vi "Get_TTL_pulse_length_at_input_2_and_start.vi"(9 "TTL pulse length to trigger start, ms":dbl=300.0, 10 "ReadStatus in":refnum<notifier>, 11 "VISA resource name":refnum<visa-resource-name>="ASRL3::INSTR") -> (0 "Start acquisition":bool, 1 "Measured TTL pulse length":dbl=0.41002368927001953, 2 "ReadStatus out":refnum<notifier>, 3 "VISA resource name out":refnum<visa-resource-name>="ASRL3::INSTR")   [LabVIEW 2016]
panel:
  out "TTL pulse start time":timestamp=timestamp(3602496054.061625 s since 1904-01-01)
  in  "TTL pulse started":bool
  out "Notifier error out":errorcluster
  out "VISA error out":errorcluster={"status"=FALSE, "code"=1073676294, "source"="VISA Read in Stream_data.vi->Get_TTL_pulse_length_at_input_2.vi"}
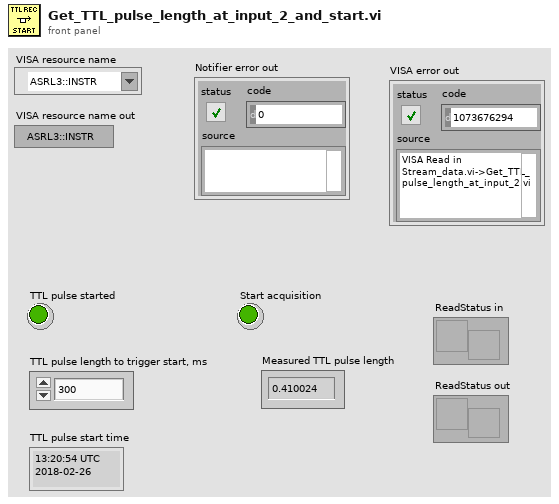
[diagram p1: front panel]
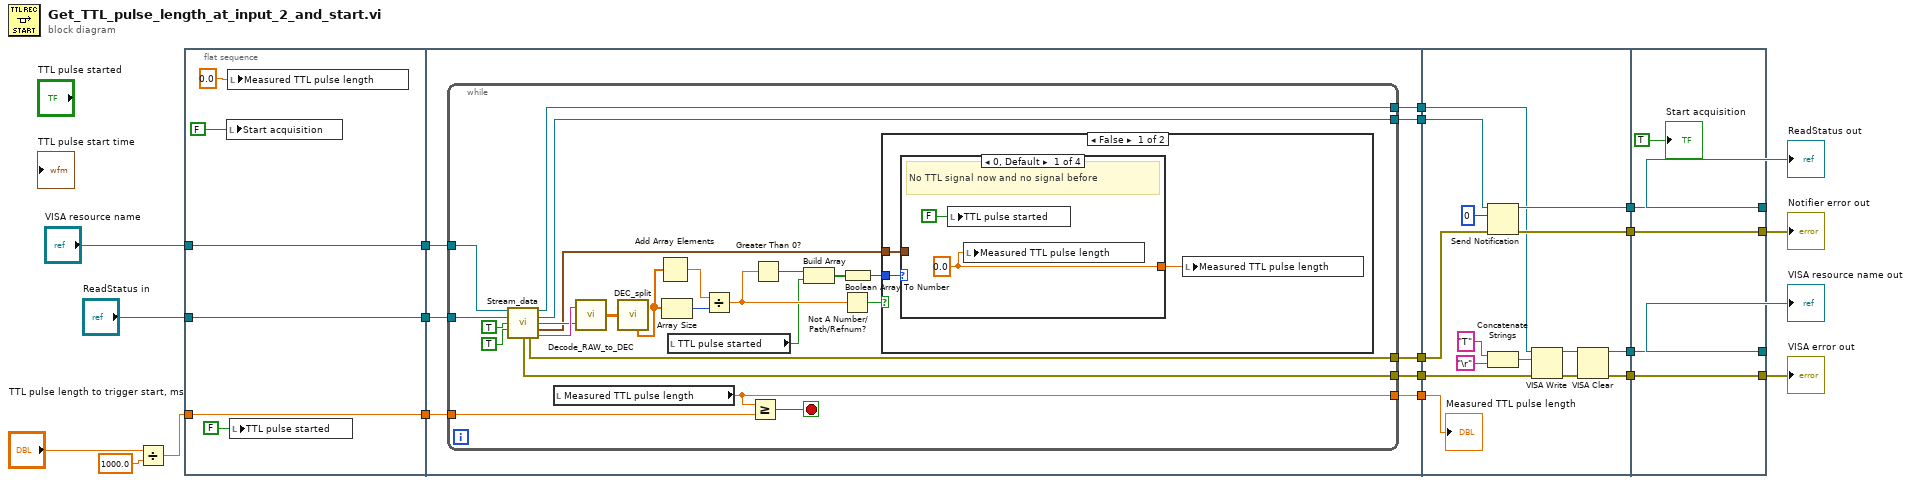
[diagram p0: block diagram]
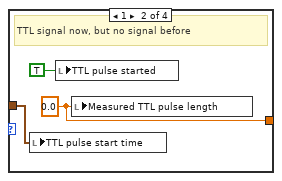
[diagram p2: hidden frame]
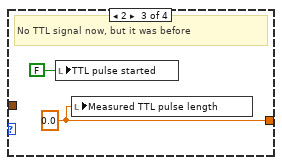
[diagram p3: hidden frame]
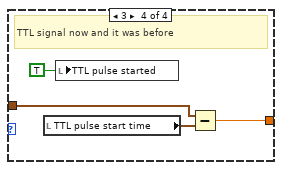
[diagram p4: hidden frame]
diagram:
  n1 = Divide(x="TTL pulse length to trigger start, ms", y=1000.0) -> (x/y=w19:dbl)
  n2 = flat-sequence {
    tunnel: w19 -> [w25]
    tunnel: "ReadStatus in" -> [w26]
    tunnel: "VISA resource name" -> [w27]
    tunnel: [w27] -> w18
    tunnel: [w26] -> w17
    tunnel: [w25] -> w16
    tunnel: w18 -> [w35]
    tunnel: w17 -> [w34]
    tunnel: w16 -> [w33]
    tunnel: [w32] -> w15
    tunnel: [w31] -> w14
    tunnel: [w30] -> w12
    tunnel: [w29] -> w10
    tunnel: [w28] -> w9
    tunnel: w15 -> [w88]
    tunnel: w14 -> [w84]
    tunnel: w12 -> [w81]
    tunnel: w10 -> [w79]
    tunnel: w9 -> [w78]
    tunnel: [w82] -> w4
    tunnel: [w80] -> w3
    tunnel: [w75] -> w2
    tunnel: [w74] -> w1
    tunnel: [w90] -> w7
    tunnel: [w91] -> w8
    tunnel: [w92] -> w11
    tunnel: [w93] -> w13
    tunnel: w4 -> [w93]
    tunnel: w3 -> [w92]
    tunnel: w2 -> [w91]
    tunnel: w1 -> [w90]
    frame #0 {
      n3 = local write "Start acquisition"(FALSE ("Start acquisition")) -> ()
      n4 = local write "Measured TTL pulse length"(0.0 ("TTL pulse length")) -> ()
      n5 = local write "TTL pulse started"(FALSE ("TTL pulse started")) -> ()
    }
    frame #1 {
      n6 = while {
        tunnel: w35 -> [w58]
        tunnel: w34 -> [w57]
        tunnel: w33 -> [w43]
        tunnel: [w41] -> w32
        tunnel: [w39] -> w31
        tunnel: [w38] -> w30
        tunnel: [w37] -> w29
        tunnel: [w36] -> w28
        stop <- w42 stop-if-true
        n7 = call "Stream_data.vi"("VISA resource name in"=w58, "ReadStatus in"=w57, "Play / Pause"=TRUE, "Read TTL status in"=TRUE ("Read TTL status")) -> ("VISA Refnum out"=w37:refnum<visa-resource-name>, "ReadStatus out"=w39:refnum<notifier>, "Read TTL status out"=w54:bool, "Current time"=w46:timestamp, "VISA error out"=w36:errorcluster, "Notifier error out"=w38:errorcluster, "read buffer"=w59:string)  [unwired: 5 in]
        n8 = local read "Measured TTL pulse length"() -> (w41:dbl)
        n9 = call "Decode_RAW_to_DEC.vi"("Read TTL status"=w54, "read buffer"=w59) -> ("DEC SGL output"=w53:sgl[][])
        n10 = call "DEC_split.vi"("Input DEC array"=w53) -> ("TTL input 2"=w50:sgl[])  [unwired: 9 out]
        n11 = Add Array Elements(numeric array=w50) -> (sum=w52:sgl)
        n12 = Array Size(array=w50) -> (size(s)=w51:i32)
        n13 = local read "TTL pulse started"() -> (w40:bool)
        n14 = Divide(x=w52, y=w51) -> (x/y=w45:sgl)
        n15 = Greater Or Equal?(x=w41, y=w43) -> (x >= y?=w42:bool)
        n16 = Greater Than 0?(x=w45) -> (x > 0?=w49:bool)
        n17 = Build Array(w49, w40) -> (w48:bool[])
        n18 = Not A Number/Path/Refnum?(number/path/refnum=w45) -> (NaN/Path/Refnum?=w44:bool)
        n19 = Boolean Array To Number(Boolean array=w48) -> (number=w47:u32)
        n20 = case shown="False" w44 {
          tunnel: w47 -> [w62 _]
          tunnel: w46 -> [w61 _]
          frame False {
            n21 = case shown="0, Default" w62 {
              tunnel: w61 -> [_ w65 _ w73]
              tunnel: [w64 w67 w69 w72] -> w60
              frame 0, Default {
                w64 = 0.0
                # "No TTL signal now and no signal before"
                n22 = local write "TTL pulse started"(FALSE ("TTL pulse started")) -> ()
                n23 = local write "Measured TTL pulse length"(w64) -> ()
              }
              frame 1 {
                w67 = 0.0
                # "TTL signal now, but no signal before"
                n24 = local write "TTL pulse start time"(w65) -> ()
                n25 = local write "TTL pulse started"(TRUE ("TTL pulse started")) -> ()
                n26 = local write "Measured TTL pulse length"(w67) -> ()
              }
              frame 2 {
                w69 = 0.0
                # "No TTL signal now, but it was before"
                n27 = local write "TTL pulse started"(FALSE ("TTL pulse started")) -> ()
                n28 = local write "Measured TTL pulse length"(w69) -> ()
              }
              frame 3 {
                # "TTL signal now and it was before"
                n29 = local read "TTL pulse start time"() -> (w71:timestamp)
                n30 = local write "TTL pulse started"(TRUE ("TTL pulse started")) -> ()
                n31 = Subtract(x=w73, y=w71) -> (x-y=w72:dbl)
              }
            }
            n32 = local write "Measured TTL pulse length"(w60) -> ()
          }
          frame True {
          }
        }
      }
    }
    frame #2 {
      n33 = Send Notification(notification=0, notifier=w84, error in (no error)=w81) -> (notifier out=w82:refnum<notifier>, error out=w80:errorcluster)
      n34 = Concatenate Strings("T" ("write buffer"), "\r") -> (w85:string)
      n35 = VISA Write(VISA resource name=w79, write buffer=w85, error in (no error)=w78) -> (VISA resource name out=w76:refnum<visa-resource-name>, error out=w77:errorcluster)  [unwired: 1 out]
      n36 = VISA Clear(VISA resource name=w76, error in (no error)=w77) -> (VISA resource name out=w74:refnum<visa-resource-name>, error out=w75:errorcluster)
      "Measured TTL pulse length" <- w88
    }
    frame #3 {
      "Start acquisition" <- TRUE ("Start acquisition")
    }
  }
  "ReadStatus out" <- w13
  "Notifier error out" <- w11
  "VISA error out" <- w8
  "VISA resource name out" <- w7
